vi "Uint64 Destroy.vi"(8 "error in (no error)":errorcluster, 11 "Uint64 DVR in":refnum<data-value>) -> (0 "error out":errorcluster)   [LabVIEW 2010, in "MDSplus.lvlib"]
uses:
  <vilib>/MDSplus/Library/MDSplus.lvlib
  <vilib>/MDSplus/Classes/Data_Class/Scalar_Class/Uint64_Class/Uint64.lvclass
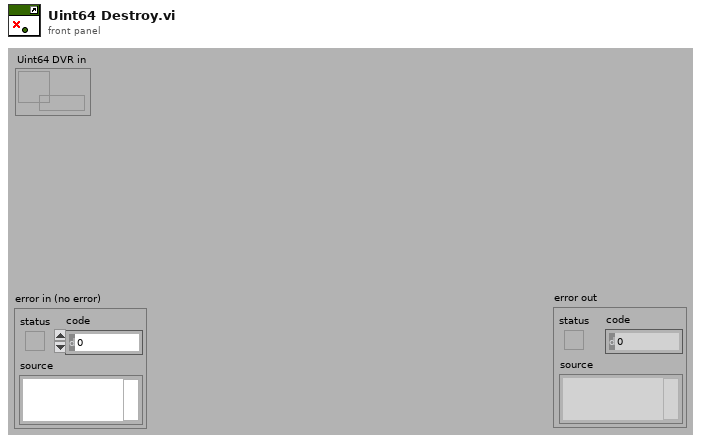
[diagram p1: front panel]
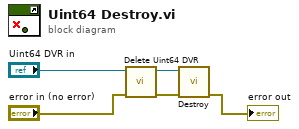
[diagram p0: block diagram]
diagram:
  n1 = call <vilib>:"Delete Uint64 DVR.vi"("error in (no error)"="error in (no error)", "Uint64 DVR in"="Uint64 DVR in") -> ("error out"=w2:errorcluster, "Uint64 out"=w3:refnum<class "Uint64.lvclass">)  [unwired: 8 in]
  n2 = call-dynamic "Destroy.vi"("error in (no error)"=w2, "Uint64 in"=w3) -> ("error out"=→"error out":errorcluster)  [unwired: 9 in]
